vi "整合读取配置文件信息头.vi"() -> (3 "Outputs":string[](array[string]))   [LabVIEW 2011]
uses:
  Global System.vi
  <vilib>/Utility/config.llb/NI_LVConfig.lvlib
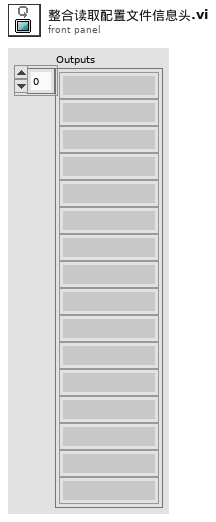
[diagram p1: front panel]
types:
  T1 = typedef "NI_LVConfig.lvlib/Config Data RefNum.ctl" = refnum<k1>
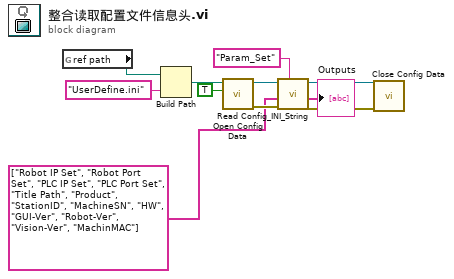
[diagram p0: block diagram]
diagram:
  n1 = global read "Global System.vi" "ref path"() -> (w11:path)
  n2 = Build Path(base path=w11, name or relative path="UserDefine.ini" ("名称或相对路径")) -> (appended path=w8:path)
  n3 = call <vilib>:"Open Config Data.vi"("create file if necessary (T)"=TRUE, "configuration file path"=w8) -> ("error out"=w6:errorcluster, "refnum"=w7:T1)  [unwired: 7 in, 1 out]
  n4 = call "Read Config_INI_String.vi"("section"="Param_Set", "error in (no error)"=w6, "Keys"=string[] ["Robot IP Set", "Robot Port Set", "PLC IP Set", "PLC Port Set", "Title Path", "Product", "StationID", "MachineSN", "HW", "GUI-Ver", "Robot-Ver", "Vision-Ver", "MachinMAC"], "refnum"=w7) -> ("error out"=w3:errorcluster, "Outputs"=→"Outputs":string[], "refnum out"=w4:T1)  [unwired: 5 in]
  n5 = call <vilib>:"Close Config Data.vi"("error in (no error)"=w3, "refnum"=w4) -> ()  [unwired: 8 in, 2 out]
